vi "配置文件保存.vi"   [LabVIEW 2016, in "斯坦道多参数.lvlib"]
uses:
  <vilib>/Utility/config.llb/NI_LVConfig.lvlib
types:
  T1 = typedef "NI_LVConfig.lvlib/Config Data RefNum.ctl" = refnum<k1>
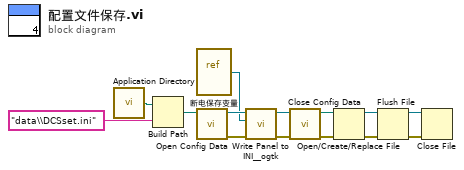
[diagram p0: block diagram]
diagram:
  n1 = call <vilib>:"Application Directory.vi"() -> ("Application Directory"=w3:path)
  n2 = Build Path(base path=w3, name or relative path="data\\DCSset.ini" ("名称或相对路径")) -> (appended path=w1:path)
  n3 = vi-ref "断电保存变量.vi"() -> (w10:refnum<vi>)
  n4 = call <vilib>:"Open Config Data.vi"("configuration file path"=w1) -> ("error out"=w13:errorcluster, "refnum"=w14:T1)  [unwired: 8 in, 1 out]
  n5 = call <userlib>:"Write Panel to INI__ogtk.vi"("error in (no error)"=w13, "VI ref"=w10, "refnum"=w14) -> ("error out"=w11:errorcluster, "refnum out"=w12:T1)  [unwired: 7 in]
  n6 = call <vilib>:"Close Config Data.vi"("error in (no error)"=w11, "refnum"=w12) -> ("error out"=w6:errorcluster, "file path"=w7:path)  [unwired: 8 in]
  n7 = Open/Create/Replace File(file path (use dialog)=w7, error in=w6) -> (refnum out=w8:refnum<file>, error out=w9:errorcluster)  [unwired: 4 in, 1 out]
  n8 = Flush File(refnum=w8, error in=w9) -> (refnum out=w4:refnum<file>, error out=w5:errorcluster)
  n9 = Close File(refnum=w4, error in=w5) -> ()  [unwired: 2 out]
